vi "Post-Process.vi"(11 "Base jettl in":refnum<class "Base jettl.lvclass">) -> ()   [LabVIEW 2021, in "jettl.lvlib" / "Base jettl.lvclass"]
uses:
  Base jettl.lvclass
  Last Ack Msg Strategy/Last Ack Msg Strategy.lvlib
  C:/git/jettl/jettl/jettl/jettl/jettl.lvclass
  C:/git/jettl/jettl/Create Msg Strategy/Create/Create.lvclass
  C:/git/jettl/jettl/jettl/Last Ack Msg Strategy/Last Ack/Last Ack.lvclass
  C:/git/jettl/jettl/Merge Error Msg Strategy/Merge Error/Merge Error.lvclass
  C:/git/jettl/jettl/Override Error Msg Strategy/Override Error/Override Error.lvclass
  C:/git/jettl/jettl/Setup Msg Strategy/Setup/Setup.lvclass
  C:/git/jettl/jettl/Teardown Msg Strategy/Teardown/Teardown.lvclass
  C:/git/jettl/jettl/jettl/Base jettl/Base jettl.lvclass
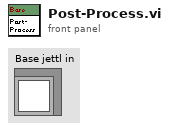
[diagram p1: front panel]
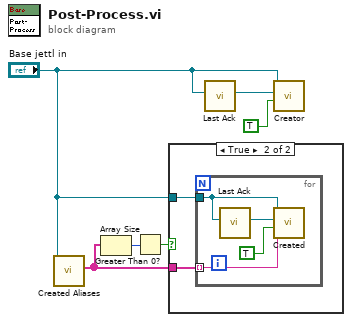
[diagram p0: block diagram]
diagram:
  n1 = call-dynamic "Created Aliases.vi"("Base jettl in"="Base jettl in") -> ("Created Aliases"=w5:string[])  [unwired: 10 in]
  n2 = Array Size(array=w5) -> (size(s)=w4:i32)
  n3 = Greater Than 0?(x=w4) -> (x > 0?=w3:bool)
  n4 = case shown="True" w3 {
    tunnel: w5 -> [_ w8]
    tunnel: "Base jettl in" -> [_ w7]
    frame False {
    }
    frame True {
      n5 = for {
        tunnel: w7 -> [w10]
        tunnel: w8 -> [w12] mode=indexing
        n6 = call "Last Ack.vi"("jettl"=w10) -> ("Msg Strategy"=w9:refnum<class "Msg Strategy.lvclass">)  [unwired: 10 in]
        n7 = call-dynamic "Created.vi"("Created Alias"=w12, "Priority?"=TRUE, "Msg Strategy"=w9, "Base jettl in"=w10) -> ()  [unwired: 7 in, 1 out]
      }
    }
  }
  n8 = call "Last Ack.vi"("jettl"="Base jettl in") -> ("Msg Strategy"=w1:refnum<class "Msg Strategy.lvclass">)  [unwired: 10 in]
  n9 = call-dynamic "Creator.vi"("Priority?"=TRUE, "Msg Strategy"=w1, "Base jettl in"="Base jettl in") -> ()  [unwired: 8 in, 1 out]
